vi "RefreshEntireTree.vi"(7 "calling VI in":refnum<vi>, 8 "error in":errorcluster, 10 "array":T1[](array[typedef]), 11 "tree ref in":refnum<vi>) -> (0 "error out":errorcluster)   [LabVIEW 2013, in "NISE_CEF_TreeControl.lvlib"]
doc: "This VI refreshes the complete tree based on the node summary"
uses:
  NISE_CEF_TreeControl.lvlib
  Node/Summary.ctl
  Node/NISE_CEF_Node.lvclass
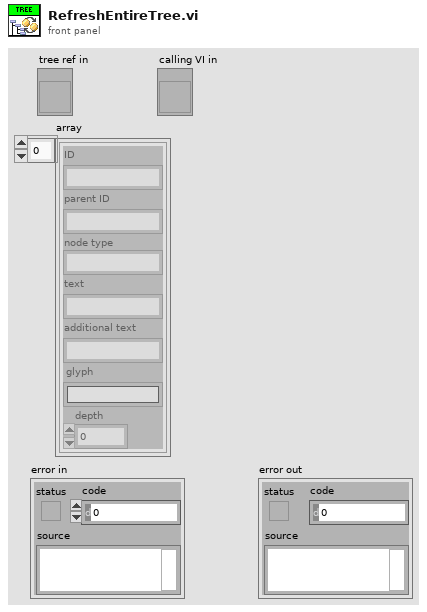
[diagram p1: front panel]
types:
  T1 = typedef "NISE_CEF_Node.lvclass/Summary.ctl" = cluster{"ID":string, "parent ID":string, "node type":string, "text":string, "additional text":string, "glyph":string, "depth":i32}
  T2 = cluster{"Left Cell String":string, "Child text":string[], "Child Tag":string, "Item Indent":i32, "Child Only?":bool, "glyph Index":i32}
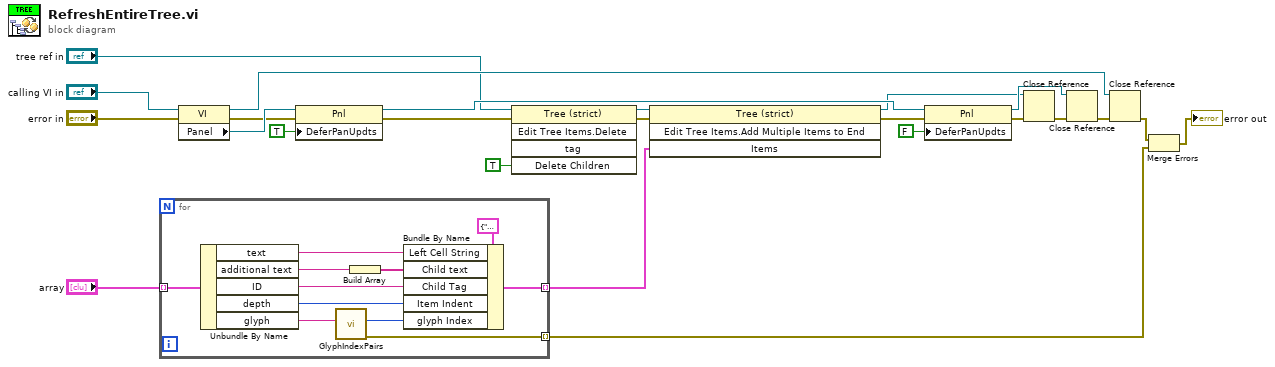
[diagram p0: block diagram]
diagram:
  n1 = for {
    tunnel: "array" -> [w35] mode=indexing
    tunnel: [w33] -> w6 mode=indexing
    tunnel: [w25] -> w1 mode=indexing
    n2 = Unbundle By Name(w35) -> ("text"=w32:string, "additional text"=w30:string, "ID"=w29:string, "depth"=w28:i32, "glyph"=w27:string)
    n3 = call "GlyphIndexPairs.vi"("glyph"=w27) -> ("error out"=w25:errorcluster, "index"=w26:i32)  [unwired: 9 in]
    n4 = Build Array(w30) -> (w31:string[])
    n5 = Bundle By Name(cluster=T2 {"Left Cell String"="", "Child text"=[], "Child Tag"="", "Item Indent"=0, "Child Only?"=FALSE, "glyph Index"=0} ("Item"), "Left Cell String"=w32, "Child text"=w31, "Child Tag"=w29, "Item Indent"=w28, "glyph Index"=w26) -> (w33:T2)
  }
  n6 = property class="VI"(reference="calling VI in", error in="error in") -> (reference out=w14:refnum<vi>, error out=w22:errorcluster, "Panel"=w23:refnum<vi>)
  n7 = property class="Pnl"(reference=w23, error in=w22, "DeferPanUpdts"=TRUE ("Defer Panel Updates")) -> (reference out=w18:refnum<vi>, error out=w7:errorcluster)
  n8 = invoke class="Tree (strict)" method="Edit Tree Items.Delete"(reference="tree ref in", error in=w7, "Delete Children"=TRUE ("Delete Children?")) -> (reference out=w9:refnum<vi>, error out=w5:errorcluster)  [unwired: 2 in, 3 out]
  n9 = invoke class="Tree (strict)" method="Edit Tree Items.Add Multiple Items to End"(reference=w9, error in=w5, "Items"=w6) -> (reference out=w8:refnum<vi>, error out=w4:errorcluster)  [unwired: 1 in, 2 out]
  n10 = property class="Pnl"(reference=w18, error in=w4, "DeferPanUpdts"=FALSE ("Defer Panel Updates")) -> (reference out=w15:refnum<vi>, error out=w17:errorcluster)
  n11 = Close Reference(reference=w8, error in (no error)=w17) -> (error out=w16:errorcluster)
  n12 = Close Reference(reference=w15, error in (no error)=w16) -> (error out=w13:errorcluster)
  n13 = Close Reference(reference=w14, error in (no error)=w13) -> (error out=w2:errorcluster)
  n14 = Merge Errors(w2, w1) -> (→"error out":errorcluster)
